vi "Send Settings.vi"(8 "error in (no error)":errorcluster, 11 "2230G in":refnum<class "2230G.lvclass">) -> (0 "error out":errorcluster, 3 "2230G out":refnum<class "2230G.lvclass">)   [LabVIEW 2018, in "2230G.lvlib" / "2230G.lvclass"]
uses:
  2230G.lvclass
  PPLs/Power Supply/Parent/Power_Supply.lvlibp/Power Supply.lvclass
  C:/Projects/LabVIEW/PPLs/Power Supply/Parent/Power_Supply.lvlibp/Power Supply.lvclass
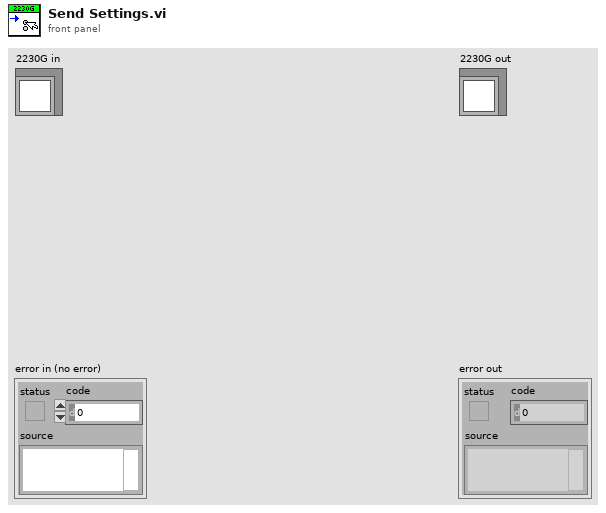
[diagram p1: front panel]
types:
  T1 = typedef "Power_Supply.lvlibp/Channel List.ctl" = enum16{"Channel 1", "Channel 2", "Channel 3", "Channel 4"}
  T2 = typedef "Power_Supply.lvlibp/Supply Settings.ctl" = cluster{"Voltage":dbl, "Current":dbl, "Output":bool}
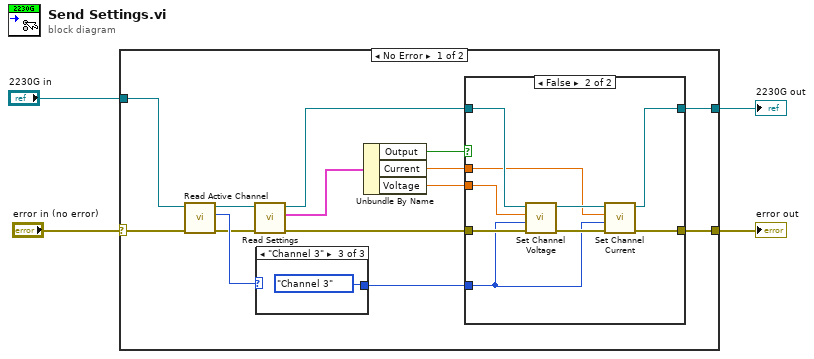
[diagram p0: block diagram]
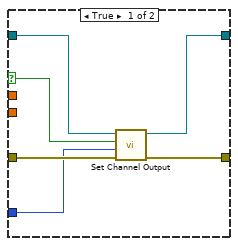
[diagram p2: hidden frame]
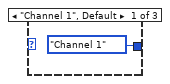
[diagram p3: hidden frame]
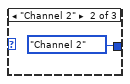
[diagram p4: hidden frame]
diagram:
  n1 = case shown="No Error" "error in (no error)" {
    selector: "error in (no error)" -> [w5 w38]
    tunnel: [w14 w38] -> w3
    tunnel: [w7 w37] -> w2
    tunnel: "2230G in" -> [w6 w37]
    frame No Error {
      n2 = call "Read Active Channel.vi"("error in (no error)"=w5, "Power Supply in"=w6) -> ("error out"=w16:errorcluster, "Active Channel"=w17:T1, "Power Supply out"=w15:refnum<class "2230G.lvclass">)  [unwired: 7 in]
      n3 = call "Read Settings.vi"("error in (no error)"=w16, "Power Supply in"=w15) -> ("error out"=w11:errorcluster, "Settings"=w18:T2, "Power Supply out"=w8:refnum<class "2230G.lvclass">)  [unwired: 7 in]
      n4 = case shown="\"Channel 3\"" w17 {
        tunnel: [enum16{"Channel 1", "Channel 2", "Channel 3"}."Channel 1" ("Channel Select") enum16{"Channel 1", "Channel 2", "Channel 3"}."Channel 2" ("Channel Select") enum16{"Channel 1", "Channel 2", "Channel 3"}."Channel 3" ("Channel Select")] -> w10
        frame "Channel 1", Default {
        }
        frame "Channel 2" {
        }
        frame "Channel 3" {
        }
      }
      n5 = Unbundle By Name(w18) -> ("Output"=w9:bool, "Current"=w13:dbl, "Voltage"=w12:dbl)
      n6 = case shown="False" w9 {
        selector: w9 -> [w24 _]
        tunnel: [w20 w25] -> w14
        tunnel: w13 -> [_ w27]
        tunnel: w12 -> [_ w31]
        tunnel: w11 -> [w23 w33]
        tunnel: w10 -> [w19 w28]
        tunnel: w8 -> [w22 w32]
        tunnel: [w21 w26] -> w7
        frame True {
          n7 = call "Set Channel Output.vi"("error in (no error)"=w23, "Channel Select"=w19, "Enable Output (T: On)"=w24, "2230G in"=w22) -> ("error out"=w20:errorcluster, "2230G out"=w21:refnum<class "2230G.lvclass">)  [unwired: 6 in]
        }
        frame False {
          n8 = call "Set Channel Voltage.vi"("error in (no error)"=w33, "Channel Select"=w28, "Voltage"=w31, "2230G in"=w32) -> ("error out"=w29:errorcluster, "2230G out"=w30:refnum<class "2230G.lvclass">)  [unwired: 6 in]
          n9 = call "Set Channel Current.vi"("error in (no error)"=w29, "Channel Select"=w28, "Current"=w27, "2230G in"=w30) -> ("error out"=w25:errorcluster, "2230G out"=w26:refnum<class "2230G.lvclass">)  [unwired: 6 in]
        }
      }
    }
    frame Error {
    }
  }
  "error out" <- w3
  "2230G out" <- w2
